vi "Line Configuration Dialog.vi"(8 "error in":errorcluster, 9 "engine configuration in":refnum<class "engine configuration.lvclass">, 10 "tag bus configurable plugin module configuration":refnum<class "Shared Memory configuration.lvclass">, 11 "Line":T3) -> (0 "error out":errorcluster, 1 "success":bool, 2 "changed":bool, 3 "Mappings out":T2)   [LabVIEW 2014, in "Shared Memory editor node.lvclass"]
doc: "A dialog for allowing a user to specify the values of a new line."
uses:
  Shared Memory editor node.lvclass
  module/configuration/Line.ctl
  <vilib>/NI/Tag Bus Module Framework/channel/TBM channel.lvclass
  Mappings.ctl
  Map.ctl
  permissions.ctl
  <vilib>/NI/Module Execution Interface/Engine Configuration/engine configuration.lvclass
  module/configuration/Shared Memory configuration.lvclass
  <vilib>/NI/Tag Bus Module Framework/channel/TBM channel.lvclass/TBM channel.ctl
  <vilib>/NI/Tag Bus/tag/tag descriptor.lvclass/tag descriptor.ctl
  <vilib>/NI/Configuration Framework/serializable configuration/NISE_CEF_serializable configuration.lvclass/NISE_CEF_serializable configuration.ctl
  <vilib>/NI/Tag Bus/tag/write tag name.vi
  <vilib>/NI/Tag Bus/tag/write data type.vi
  <vilib>/NI/Tag Bus Module Framework/channel/Write channel classification.vi
  <vilib>/NI/Configuration Framework/serializable configuration/Read UID.vi
  <vilib>/NI/Tag Bus Module Framework/channel/Read channel classification.vi
  <vilib>/NI/Tag Bus/tag/read data type.vi
  <vilib>/Utility/LVClass/Get LV Class Name.vi
  <vilib>/NI/Configuration Framework/error generator/NISE_error generator.vi
  <vilib>/NI/Tag Bus/tag/tag descriptor.lvclass
  <vilib>/NI/DCAF UI Toolkit/Controls/DCAF UI Elements.lvlib
panel:
  out "errors":string
  in  "Access Type":T1=enum."Read from Memory"
  in  "Tag":i32(listbox)
  in  "Data Type":i32(listbox)
  in  "Channel Name":string
  in  "cancel":bool
  in  "ok":bool
  # "#CodeRecommended Add implementation details here. For example, a shared variable URL."
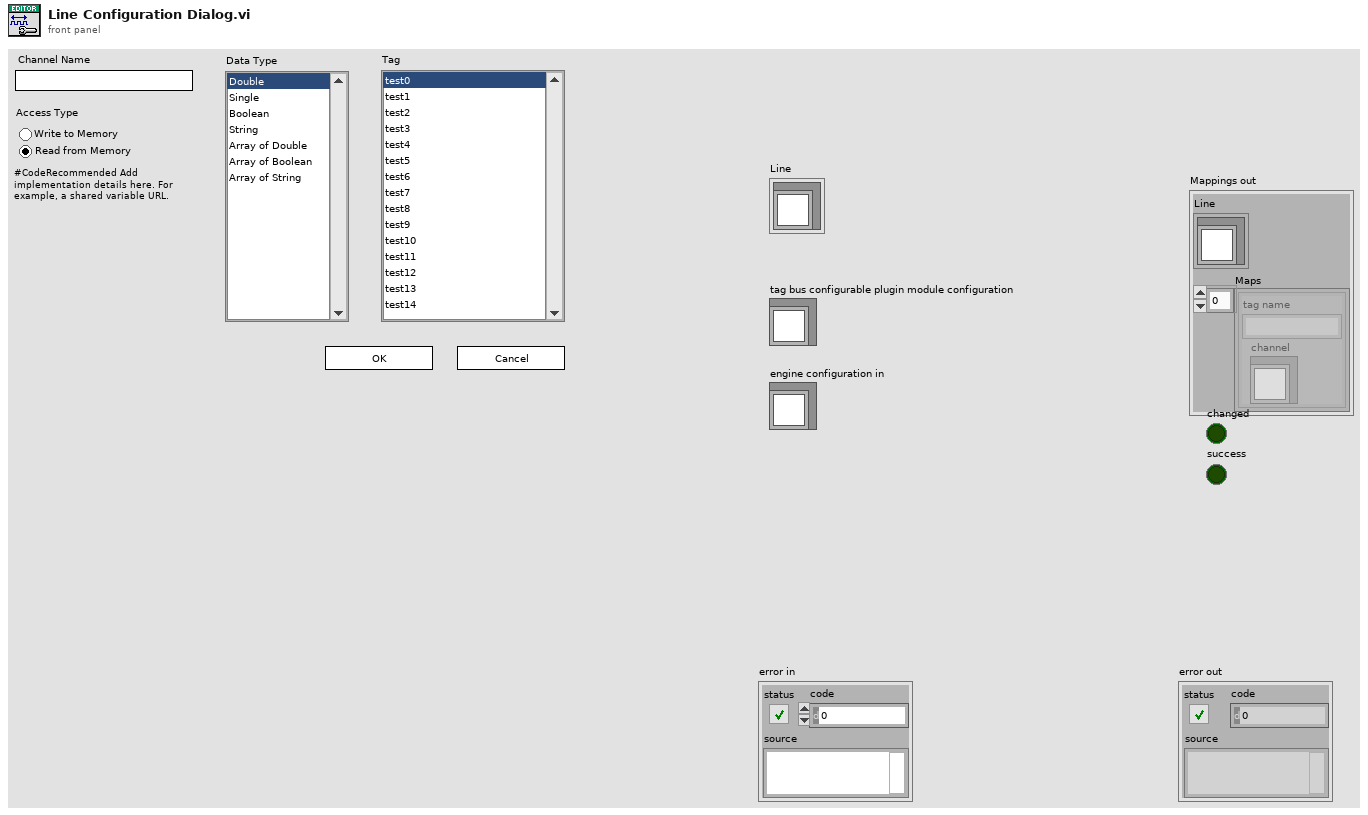
[diagram p1: front panel]
types:
  T1 = typedef "Shared Memory editor node.lvclass/permissions.ctl" = enum32{"Write to Memory", "Read from Memory"}
  T2 = typedef "Shared Memory editor node.lvclass/Mappings.ctl" = cluster{"Line":T3, "Maps":T4[]}
  T3 = typedef "Shared Memory configuration.lvclass/Line.ctl" = cluster{"channel":refnum<class "TBM channel.lvclass">}
  T4 = typedef "Shared Memory editor node.lvclass/Map.ctl" = cluster{"channel":refnum<class "TBM channel.lvclass">, "tag name":string}
  T5 = typedef "tag bus.lvlib/tag descriptor.lvclass/Data Type.ctl" = enum16{"Double", "Single", "I64", "I32", "I16", "I8", "U64", "U32", "U16", "U8", "Boolean", "String", "Array of Double", "Array of Single", "Array of I64", "Array of I32", "Array of I16", "Array of I8", "Array of U64", "Array of U32", "Array of U16", "Array of U8", "Array of Boolean", "Array of String"}
  T6 = typedef "TBM channel.lvclass/channel classification.ctl" = enum16{"input data", "output data", "processing parameter", "processing result"}
  T7 = enum8{"Enabled", "Disabled", "Disabled and Grayed Out"}
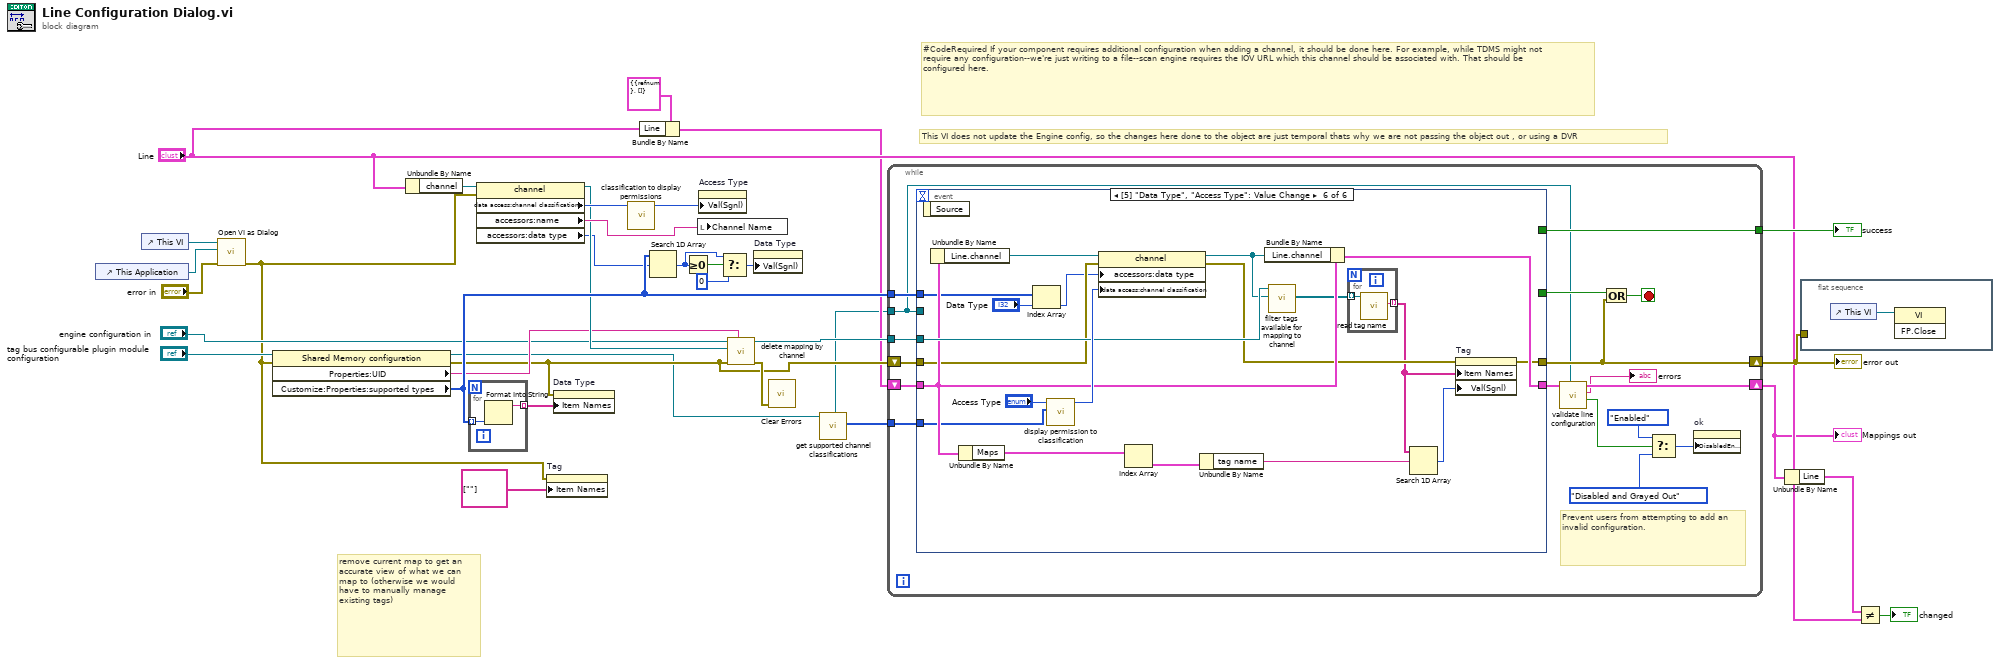
[diagram p0: block diagram]
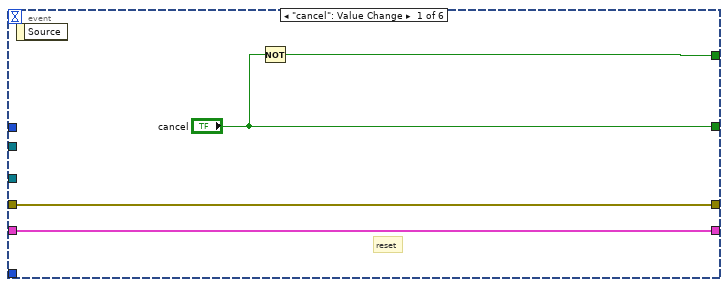
[diagram p2: hidden frame]
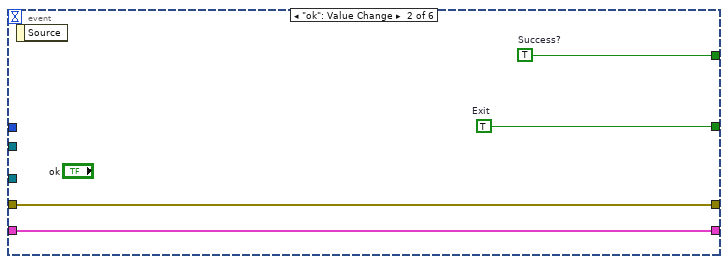
[diagram p3: hidden frame]
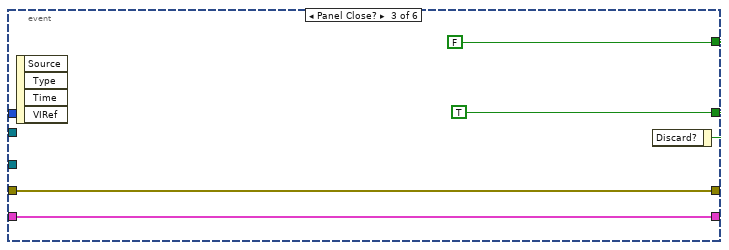
[diagram p4: hidden frame]
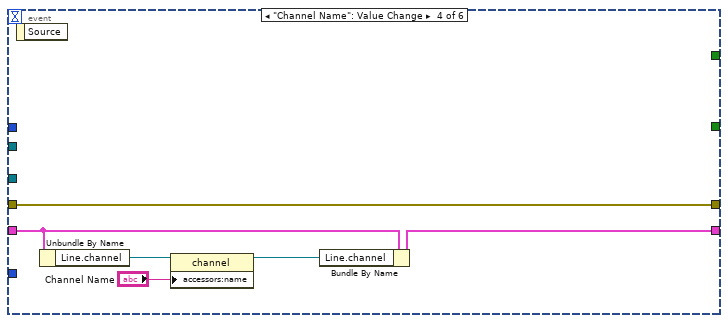
[diagram p5: hidden frame]
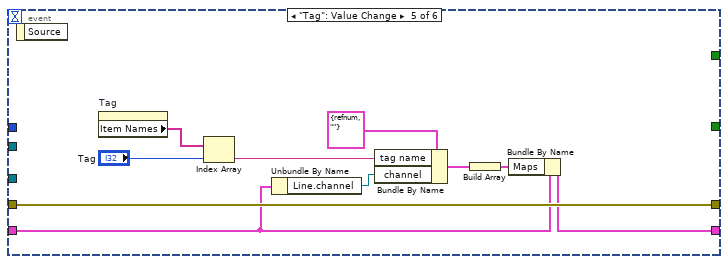
[diagram p6: hidden frame]
diagram:
  # "This VI does not update the Engine config, so the changes here done to the object are just temporal thats why we are not passing the object out , or using a DVR"
  # "remove current map to get an accurate view of what we can map to (otherwise we would have to manually manage existing tags)"
  # "#CodeRequired If your component requires additional configuration when adding a channel, it should be done here. For example, while TDMS might not require any configuration--we're just writing to a file--scan engine requires the IOV URL which this channel should be associated with. That should be configured here."
  n1 = control-ref of="This Application"() -> (w6:refnum<vi>)
  n2 = control-ref of="This VI"() -> (w7:refnum<vi>)
  n3 = call <vilib>:"Open VI as Dialog.vi"("error in (no error)"="error in", "This Application"=w6, "VI in"=w7) -> ("error out"=w4:errorcluster)  [unwired: 8 in]
  n4 = property class="Shared Memory configuration"(reference="tag bus configurable plugin module configuration", error in=w4) -> (reference out=w3:refnum<class "Shared Memory configuration.lvclass">, error out=w14:errorcluster, "Properties:UID"=w25:string, "Customize:Properties:supported types"=w31:T5[])
  n5 = Unbundle By Name("Line") -> ("channel"=w27:refnum<class "TBM channel.lvclass">)
  n6 = for {
    tunnel: w31 -> [w36] mode=indexing
    tunnel: [w35] -> w24 mode=indexing
    n7 = Format Into String(w36) -> (resulting string=w35:string)  [unwired: 3 in, 1 out]
  }
  n8 = property class="channel"(reference=w27, error in=w4) -> (reference out=w26:refnum<class "TBM channel.lvclass">, "data access:channel classification"=w29:T6, "accessors:name"=w28:string, "accessors:data type"=w17:T5)  [unwired: 1 out]
  n9 = property on="Tag" class="LstBox (strict)"(error in=w4, "Item Names"=string[] [""]) -> ()  [unwired: 1 in, 2 out]
  n10 = property on="Data Type" class="LstBox (strict)"(error in=w14, "Item Names"=w24) -> ()  [unwired: 1 in, 2 out]
  n11 = call "classification to display permissions.vi"("channel classification"=w29) -> ("permissions"=w18:T1)  [unwired: 10 in]
  n12 = Bundle By Name(cluster=T2 {"Line"={"channel"=refnum}, "Maps"=[]} ("Mappings out"), "Line"="Line") -> (w10:T2)
  n13 = Search 1D Array(1D array=w31, element=w17) -> (index of element=w22:i32)  [unwired: 1 in]
  n14 = Greater Or Equal To 0?(x=w22) -> (x >= 0?=w23:bool)
  n15 = local write "Channel Name"(w28) -> ()
  n16 = property on="Access Type" class="RadioBtnsControl (strict)"("Val(Sgnl)"=w18) -> ()  [unwired: 2 in, 2 out]
  n17 = Select(t=w22, s=w23, f=0) -> (s? t:f=w20:i32)
  n18 = call <vilib>:"delete mapping by channel.vi"("owner ID"=w25, "error in"=w14, "channel"=w26, "engine configuration in"="engine configuration in") -> ("error out"=w16:errorcluster, "engine configuration out"=w32:refnum<class "engine configuration.lvclass">)  [unwired: 6 in]
  n19 = property on="Data Type" class="LstBox (strict)"("Val(Sgnl)"=w20) -> ()  [unwired: 2 in, 2 out]
  n20 = call <vilib>:"Clear Errors.vi"("error in (no error)"=w16) -> ()  [unwired: 5 in, 2 out]
  n21 = call-dynamic "get supported channel classifications.vi"("module configuration in"=w3) -> ("supported classes"=w1:T6[], "module configuration out"=w2:refnum<class "Shared Memory configuration.lvclass">)  [unwired: 8 in, 1 out]
  n22 = while {
    shift-right: [w45] -> w30
    shift-left: w14 -> [w52]
    tunnel: [w51] -> w34
    shift-right: [w46] -> w8
    shift-left: w10 -> [w48]
    tunnel: w32 -> [w53]
    tunnel: w2 -> [w38]
    tunnel: w31 -> [w40]
    tunnel: w1 -> [w37]
    stop <- w49 stop-if-true
    # "Prevent users from attempting to add an invalid configuration."
    n23 = event shown="[5] \"Data Type\", \"Access Type\": Value Change" {
      selector: _ -> [_ _ _ _ _ _]
      dyn-events: _ -> [_ _ _ _ _ _]
      timeout: _ -> [_ _ _ _ _ _]
      tunnel: w53 -> [_ _ _ _ _ w99]
      tunnel: w52 -> [w57 w61 w65 w71 w81 w93]
      tunnel: [w57 w61 w65 w71 w81 w88] -> w45
      tunnel: [w56 w58 FALSE _ _ _] -> w51
      tunnel: ["cancel" w59 w63 _ _ _] -> w50
      tunnel: w48 -> [w54 w60 w62 w69 w75 w97]
      tunnel: [w54 w60 w62 w70 w72 w96] -> w47
      tunnel: w38 -> [_ _ _ _ _ _]
      tunnel: w40 -> [_ _ _ _ _ w92]
      tunnel: w37 -> [_ _ _ _ _ w82]
      event "cancel": Value Change {
        # "reset"
        n24 = event-data() -> ()  [unwired: 1 in, 1 out]
        n25 = Not(x="cancel") -> (.not. x?=w56:bool)
      }
      event "ok": Value Change {
        w58 = TRUE  # Success?
        w59 = TRUE  # Exit
        n26 = event-data() -> ()  [unwired: 1 in, 1 out]
      }
      event Panel Close? {
        w63 = TRUE ("cancel")
        n27 = event-data() -> ()  [unwired: 1 in, 4 out]
        n28 = event-data("Discard?"=w63) -> ()  [unwired: 1 in, 1 out]
      }
      event "Channel Name": Value Change {
        n29 = event-data() -> ()  [unwired: 1 in, 1 out]
        n30 = Unbundle By Name(w69) -> ("Line.channel"=w68:refnum<class "TBM channel.lvclass">)
        n31 = property class="channel"(reference=w68, "accessors:name"="Channel Name") -> (reference out=w67:refnum<class "TBM channel.lvclass">)  [unwired: 1 in, 1 out]
        n32 = Bundle By Name(cluster=w69, "Line.channel"=w67) -> (w70:T2)
      }
      event "Tag": Value Change {
        n33 = event-data() -> ()  [unwired: 1 in, 1 out]
        n34 = property on="Tag" class="LstBox (strict)"() -> ("Item Names"=w79:string[])  [unwired: 2 in, 2 out]
        n35 = Index Array(array=w79, index="Tag") -> (element=w78:string)
        n36 = Unbundle By Name(w75) -> ("Line.channel"=w76:refnum<class "TBM channel.lvclass">)
        n37 = Bundle By Name(cluster=T4 {"channel"=refnum, "tag name"=""} ("Map"), "tag name"=w78, "channel"=w76) -> (w74:T4)
        n38 = Build Array(w74) -> (w73:T4[])
        n39 = Bundle By Name(cluster=w75, "Maps"=w73) -> (w72:T2)
      }
      event "Data Type": Value Change {
        n40 = event-data() -> ()  [unwired: 1 in, 1 out]
        n41 = Unbundle By Name(w97) -> ("Line.channel"=w101:refnum<class "TBM channel.lvclass">)
        n42 = Unbundle By Name(w97) -> ("Maps"=w85:T4[])
        n43 = Index Array(array=w92, index="Data Type") -> (element=w90:T5)
        n44 = call "display permission to classification.vi"("supported classes"=w82, "display permissions"="Access Type") -> ("channel classification"=w100:T6)  [unwired: 9 in]
        n45 = property class="channel"(reference=w101, error in=w93, "accessors:data type"=w90, "data access:channel classification"=w100) -> (reference out=w98:refnum<class "TBM channel.lvclass">, error out=w89:errorcluster)
        n46 = Index Array(array=w85) -> (element=w84:T4)  [unwired: 1 in]
        n47 = Unbundle By Name(w84) -> ("tag name"=w83:string)
        n48 = Bundle By Name(cluster=w97, "Line.channel"=w98) -> (w96:T2)
        n49 = call-dynamic "filter tags available for mapping to channel.vi"("channel to map to"=w98, "engine configuration in"=w99) -> ("filtered tags"=w95:refnum<class "tag descriptor.lvclass">[])  [unwired: 8 in, 1 out]
        n50 = for {
          tunnel: w95 -> [w103] mode=indexing
          tunnel: [w102] -> w87 mode=indexing
          n51 = call <vilib>:"read tag name.vi"("system tag in"=w103) -> ("name"=w102:string)  [unwired: 8 in, 2 out]
        }
        n52 = Search 1D Array(1D array=w87, element=w83) -> (index of element=w86:i32)  [unwired: 1 in]
        n53 = property on="Tag" class="LstBox (strict)"(error in=w89, "Item Names"=w87, "Val(Sgnl)"=w86) -> (error out=w88:errorcluster)  [unwired: 1 in, 1 out]
      }
    }
    n54 = call "validate line configuration.vi"("Module Config"=w38, "Mappings in"=w47) -> ("valid?"=w44:bool, "errors"=→"errors":string, "Mappings out"=w46:T2)  [unwired: 7 in]
    n55 = Compound Arithmetic op=OR(w50, w45) -> (w49:bool)
    n56 = Select(t=T7."Enabled" ("Disabled"), s=w44, f=T7."Disabled and Grayed Out") -> (s? t:f=w41:T7)
    n57 = property on="ok" class="Bool"("DisabledEnum"=w41) -> ()  [unwired: 2 in, 2 out]
  }
  "error out" <- w30
  "success" <- w34
  "Mappings out" <- w8
  n58 = Unbundle By Name(w8) -> ("Line"=w9:T3)
  n59 = flat-sequence {
    tunnel: w30 -> [_]
    frame #0 {
      n60 = control-ref of="This VI"() -> (w104:refnum<vi>)
      n61 = invoke class="VI" method="FP.Close"(reference=w104) -> ()  [unwired: 2 in, 3 out]
    }
  }
  n62 = Not Equal?(x=w9, y="Line") -> (x != y?=→"changed":bool)
